vi "Pulse Measurements 1 chan.vi"(5 "export mode":u16(ring) items=["all", "no period and duty cycle"], 6 "percent level settings":T2={"method"=enum."auto select", "histogram size"=256, "histogram method"=enum."mode", "reserved"=1.0} {"reserved" format="%0.2f"}, 7 "pulse number (1)":i32=1 min=1, 8 "error in (no error)":errorcluster, 9 "reference levels":T3={"high ref level"=90.0, "mid ref level"=50.0, "low ref level"=10.0, "ref units"=1} {"ref units" items=["absolute", "percent"]; "high ref level" format="%0.2f"; "low ref level" format="%0.2f"; "mid ref level" format="%0.2f"}, 10 "polarity (high)":u16(ring)=1 items=["low pulse", "high pulse"], 11 "signal in":waveform(dbl)={"t0"=timestamp(0 s since 1904-01-01), "dt"=0.0, "Y"=[]}) -> (0 "error out":errorcluster, 1 "duty cycle":dbl format="%.2g", 2 "pulse duration":dbl format="%.2g", 3 "period":dbl format="%.2g", 4 "measurement info":T1 {"ref levels"."ref units" items=["absolute", "relative"]; "ref levels"."high ref level" format="%.2p"; "ref levels"."low ref level" format="%.2p"; "ref levels"."mid ref level" format="%.2p"; "pulse center" format="%.2p"})   [LabVIEW 2020, in "NI_MAPro.lvlib"]
doc: "Accepts a periodic waveform or an array of periodic waveforms and returns the <B>period</B>, <B>pulse duration</B> (pulse width), <B>duty cycle</B> (duty factor), and <B>pulse center</B> of a selected pulse and period. Wire data to the <B>signal in</B> input to determine the polymorphic instance to use or manually select the instance."
uses:
  NI_MAPro.lvlib
  NI_MABase.lvlib
  <resource>/lvanlys.dll
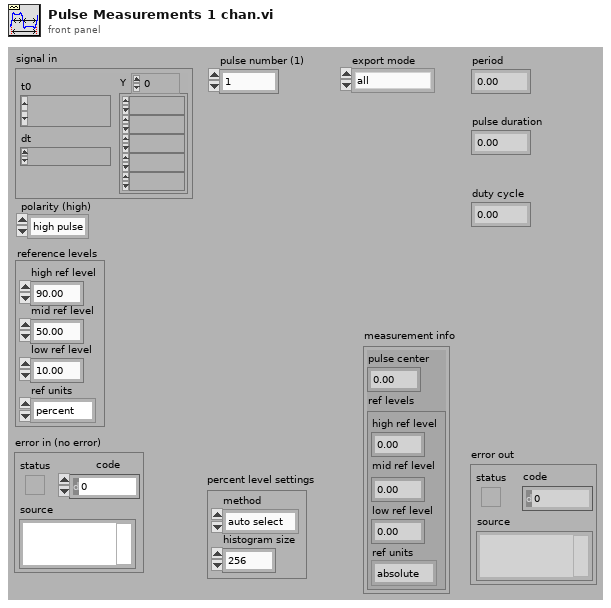
[diagram p1: front panel]
types:
  T1 = cluster{"pulse center":dbl, "ref levels":cluster{"high ref level":dbl, "mid ref level":dbl, "low ref level":dbl, "ref units":u16}}
  T2 = cluster{"method":enum32{"histogram", "peak", "auto select"}, "histogram size":i32, "histogram method":enum16{"mode"}, "reserved":dbl}
  T3 = cluster{"high ref level":dbl, "mid ref level":dbl, "low ref level":dbl, "ref units":u16}
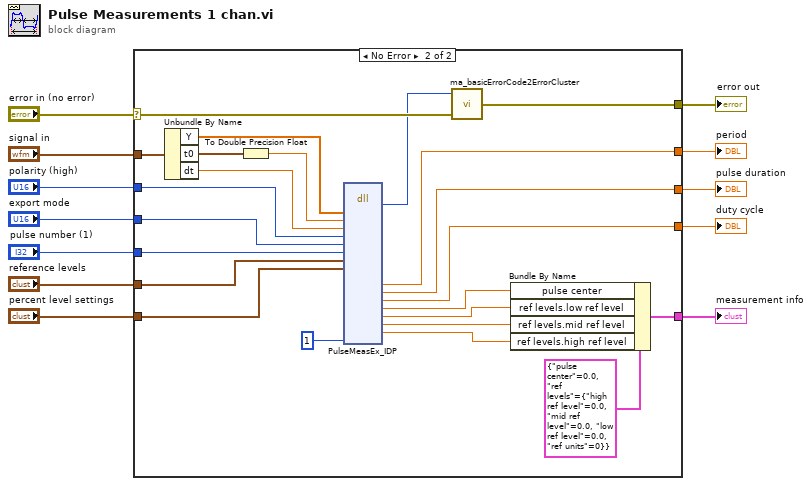
[diagram p0: block diagram]
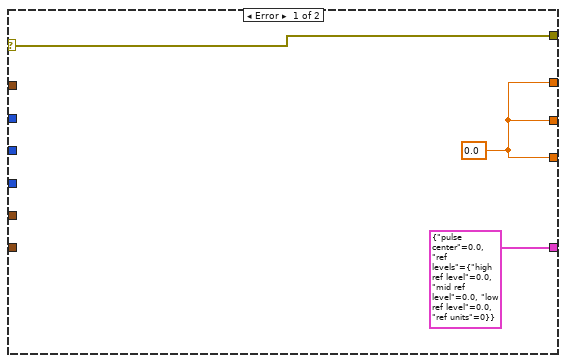
[diagram p2: hidden frame]
diagram:
  n1 = case shown="No Error" "error in (no error)" {
    selector: "error in (no error)" -> [w15 w37]
    tunnel: "polarity (high)" -> [_ w32]
    tunnel: "reference levels" -> [_ w34]
    tunnel: "percent level settings" -> [_ w35]
    tunnel: "pulse number (1)" -> [_ w33]
    tunnel: "signal in" -> [_ w38]
    tunnel: [w15 w28] -> w6
    tunnel: [w14 w29] -> w5
    tunnel: [w14 w30] -> w4
    tunnel: [w14 w31] -> w3
    tunnel: [T1 {"pulse center"=0.0, "ref levels"={"high ref level"=0.0, "mid ref level"=0.0, "low ref level"=0.0, "ref units"=0}} ("measurement info") w36] -> w2
    tunnel: "export mode" -> [_ w27]
    frame Error {
      w14 = 0.0 ("result")
    }
    frame No Error {
      n2 = Unbundle By Name(w38) -> ("Y"=w26:dbl[], "t0"=w24:timestamp, "dt"=w22:dbl)
      n3 = To Double Precision Float(number=w24) -> (double precision float=w23:dbl)
      n4 = dll-call lib="C:/Program Files (x86)/National Instruments/LabVIEW 2020/resource/lvanlys.*" fn="PulseMeasEx_IDP"("xH"=w26, "Xo"=w23, "dx"=w22, "polarity"=w32, "export_mode"=w27, "pulseNum"=w33, "refLevel"=w34, "percentLevel"=w35, "newAlgorithm"=1) -> ("return type"=w16:i32, "period"=w29:dbl, "pulseDuration"=w30:dbl, "dutyCycle"=w31:dbl, "pulseCenter"=w18:dbl, "lowRefLevel"=w19:dbl, "midRefLevel"=w20:dbl, "highRefLevel"=w21:dbl)  [unwired: 12 in, 11 out]
      n5 = call "ma_basicErrorCode2ErrorCluster.vi"("error in (no error)"=w37, "Error Code"=w16) -> ("error out"=w28:errorcluster)  [unwired: 1 in]
      n6 = Bundle By Name(cluster=T1 {"pulse center"=0.0, "ref levels"={"high ref level"=0.0, "mid ref level"=0.0, "low ref level"=0.0, "ref units"=0}} ("measurement info"), "pulse center"=w18, "ref levels.low ref level"=w19, "ref levels.mid ref level"=w20, "ref levels.high ref level"=w21) -> (w36:T1)
    }
  }
  "period" <- w5
  "pulse duration" <- w4
  "duty cycle" <- w3
  "error out" <- w6
  "measurement info" <- w2
